vi "toml_load_value.vi"(8 "error in (no error)":errorcluster, 9 "offset (0)":i32, 11 "toml":string) -> (0 "error out":errorcluster, 2 "remaining string":string, 3 "value":string)   [LabVIEW 2017]
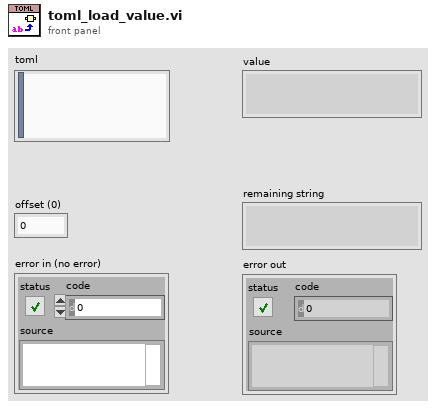
[diagram p1: front panel]
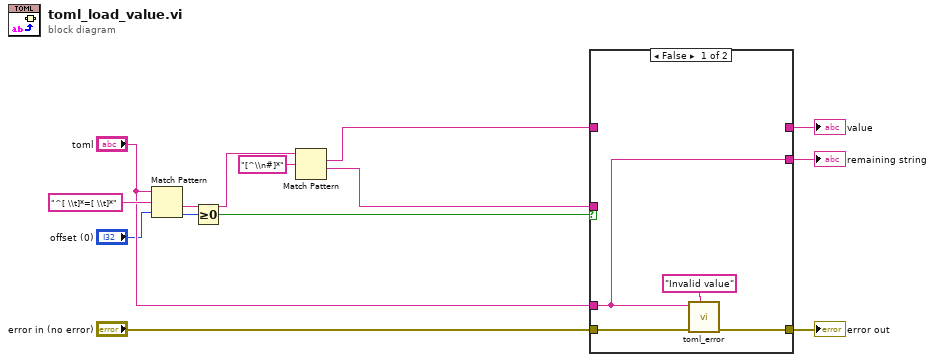
[diagram p0: block diagram]
diagram:
  n1 = Match Pattern(string="toml", regular expression="^[ \\t]*=[ \\t]*", offset (0)="offset (0)") -> (after substring=w3:string, offset past match=w7:i32)  [unwired: 2 out]
  n2 = Greater Or Equal To 0?(x=w7) -> (x >= 0?=w6:bool)
  n3 = Match Pattern(string=w3, regular expression="[^\\n#]*") -> (match substring=w1:string, after substring=w2:string)  [unwired: 1 in, 2 out]
  n4 = case shown="False" w6 {
    tunnel: "error in (no error)" -> [w17 w20]
    tunnel: [w16 w20] -> w12
    tunnel: [w14 w19] -> w11
    tunnel: "toml" -> [w14 _]
    tunnel: w2 -> [_ w19]
    tunnel: w1 -> [_ w18]
    tunnel: [_ w18] -> w5
    frame False {
      n5 = call "toml_error.vi"("message"="Invalid value", "error in (no error)"=w17, "toml"=w14) -> ("error out"=w16:errorcluster)  [unwired: 8 in]
    }
    frame True {
    }
  }
  "error out" <- w12
  "remaining string" <- w11
  "value" <- w5
